vi "9701 Missing mapping at index for Communication Parameter at index--error.vi"(8 "error in":errorcluster, 10 "Com Pam Index":u16, 11 "Mapping Index":u16) -> (0 "error out":errorcluster)   [LabVIEW 2024, in "PDO Grid.lvlib"]
uses:
  PDO Grid.lvlib
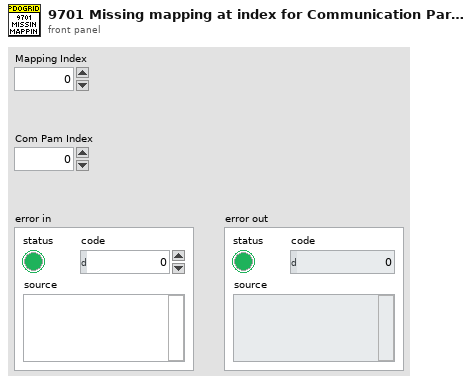
[diagram p1: front panel]
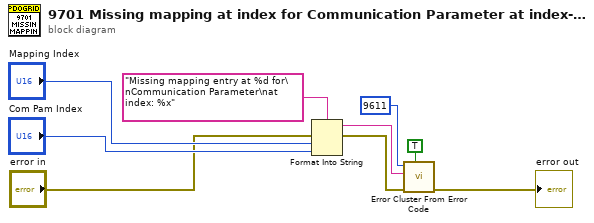
[diagram p0: block diagram]
diagram:
  n1 = Format Into String(format string="Missing mapping entry at %d for\nCommunication Parameter\nat index: %x", error in="error in", "Mapping Index", "Com Pam Index") -> (resulting string=w8:string, error out=w2:errorcluster)  [unwired: 1 in]
  n2 = call <vilib>:"Error Cluster From Error Code.vi"("show call chain? (False)"=TRUE, "error in (no error)"=w2, "error message (\"\")"=w8, "error code (0)"=9611) -> ("error out"=→"error out":errorcluster)  [unwired: 5 in]
